vi "MeasureDarkCurrentSimulation.vi"() -> (2 "Amplifier Error":errorcluster)   [LabVIEW 2017]
uses:
  AmplifierSim.lvclass
  MultimeterSim.lvclass
panel:
  out "Final voltage":dbl
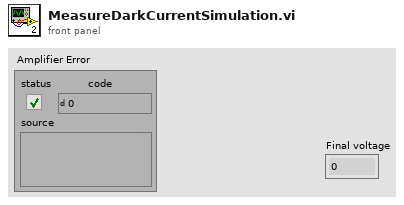
[diagram p1: front panel]
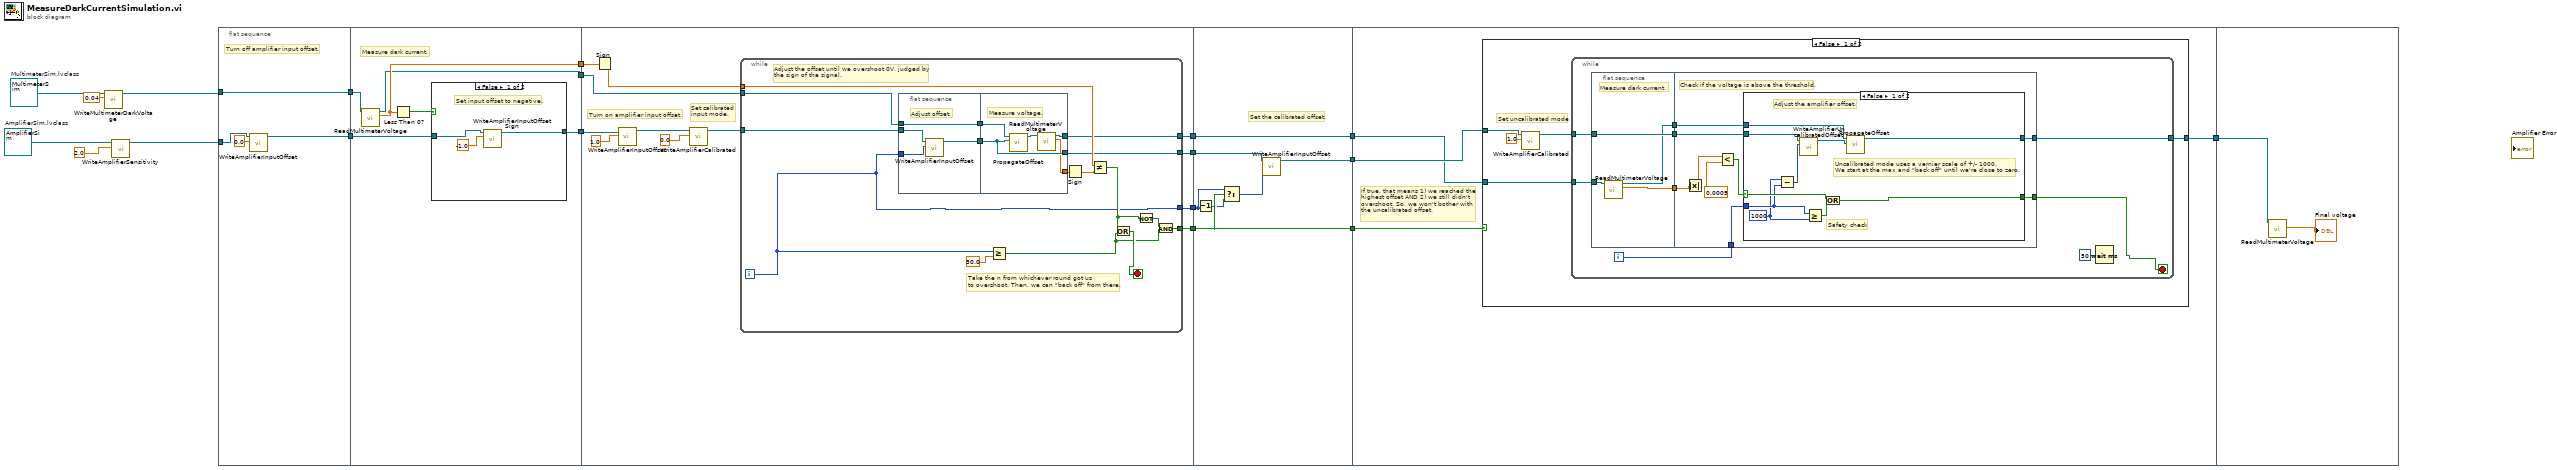
[diagram p0: block diagram]
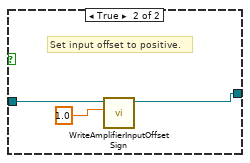
[diagram p2: hidden frame]
diagram:
  w6 = refnum<class "MultimeterSim.lvclass"> refnum  # MultimeterSim.lvclass
  w3 = refnum<class "AmplifierSim.lvclass"> refnum  # AmplifierSim.lvclass
  n1 = call-dynamic "WriteMultimeterDarkVoltage.vi"("Dark Voltage"=0.04, "MultimeterSim in"=w6) -> ("MultimeterSim out"=w5:refnum<class "MultimeterSim.lvclass">)  [unwired: 8 in, 1 out]
  n2 = call-dynamic "WriteAmplifierSensitivity.vi"("Sensitivity"=2.0, "AmplifierSim in"=w3) -> ("AmplifierSim out"=w1:refnum<class "AmplifierSim.lvclass">)  [unwired: 8 in, 1 out]
  n3 = flat-sequence {
    tunnel: w1 -> [w22]
    tunnel: [w21] -> w15
    tunnel: w5 -> [w21]
    tunnel: [w20] -> w14
    tunnel: [w27] -> w19
    tunnel: w15 -> [w28]
    tunnel: w14 -> [w26]
    tunnel: [w25] -> w13
    tunnel: [w24] -> w12
    tunnel: w19 -> [w47]
    tunnel: [w45] -> w18
    tunnel: [w44] -> w16
    tunnel: w13 -> [w43]
    tunnel: w12 -> [w38]
    tunnel: [w37] -> w11
    tunnel: [w36] -> w8
    tunnel: w18 -> [w73]
    tunnel: [w76] -> w17
    tunnel: w16 -> [w76]
    tunnel: w11 -> [w79]
    tunnel: [w78] -> w10
    tunnel: [w77] -> w9
    tunnel: w8 -> [w77]
    tunnel: w17 -> [w83]
    tunnel: w10 -> [w82]
    tunnel: w9 -> [w81]
    tunnel: [w80] -> w7
    tunnel: w7 -> [w122]
    frame #0 {
      # "Turn off amplifier input offset."
      n4 = call-dynamic "WriteAmplifierInputOffset.vi"("Input Offset"=0.0, "AmplifierSim in"=w22) -> ("AmplifierSim out"=w20:refnum<class "AmplifierSim.lvclass">)  [unwired: 8 in, 1 out]
    }
    frame #1 {
      # "Measure dark current."
      n5 = call-dynamic "ReadMultimeterVoltage.vi"("MultimeterSim in"=w28) -> ("Voltage"=w27:dbl, "MultimeterSim out"=w24:refnum<class "MultimeterSim.lvclass">)  [unwired: 8 in, 1 out]
      n6 = Less Than 0?(x=w27) -> (x < 0?=w29:bool)
      n7 = case shown="False" w29 {
        tunnel: w26 -> [w31 w35]
        tunnel: [w30 w33] -> w25
        frame False {
          # "Set input offset to negative."
          n8 = call-dynamic "WriteAmplifierInputOffsetSign.vi"("Input Offset Sign"=-1.0, "AmplifierSim in"=w31) -> ("AmplifierSim out"=w30:refnum<class "AmplifierSim.lvclass">)  [unwired: 8 in, 1 out]
        }
        frame True {
          # "Set input offset to positive."
          n9 = call-dynamic "WriteAmplifierInputOffsetSign.vi"("Input Offset Sign"=1.0, "AmplifierSim in"=w35) -> ("AmplifierSim out"=w33:refnum<class "AmplifierSim.lvclass">)  [unwired: 8 in, 1 out]
        }
      }
    }
    frame #2 {
      # "Set calibrated \ninput mode."
      # "Turn on amplifier input offset."
      n10 = Sign(1:w47) -> (0:w46:dbl)
      n11 = call-dynamic "WriteAmplifierInputOffset.vi"("Input Offset"=1.0, "AmplifierSim in"=w43) -> ("AmplifierSim out"=w40:refnum<class "AmplifierSim.lvclass">)  [unwired: 8 in, 1 out]
      n12 = call-dynamic "WriteAmplifierCalibrated.vi"("Calibrated"=0.0, "AmplifierSim in"=w40) -> ("AmplifierSim out"=w39:refnum<class "AmplifierSim.lvclass">)  [unwired: 8 in, 1 out]
      n13 = while {
        tunnel: w46 -> [w61]
        tunnel: [w48] -> w45
        tunnel: [w56] -> w44
        tunnel: w39 -> [w55]
        tunnel: w38 -> [w53]
        tunnel: [w51] -> w37
        tunnel: [w50] -> w36
        i -> [w48]
        stop <- w60 stop-if-true
        # "Take the n from whichever round got us \nto overshoot. Then, we can \"back off\" from there."
        # "Adjust the offset until we overshoot 0V, judged by\nthe sign of the signal."
        n14 = flat-sequence {
          tunnel: w48 -> [w66]
          tunnel: w55 -> [w67]
          tunnel: [w65] -> w54
          tunnel: w53 -> [w64]
          tunnel: [w64] -> w52
          tunnel: w54 -> [w71]
          tunnel: w52 -> [w72]
          tunnel: [w71] -> w51
          tunnel: [w68] -> w50
          tunnel: [w70] -> w49
          frame #0 {
            # "Adjust offset."
            n15 = call-dynamic "WriteAmplifierInputOffset.vi"("Input Offset"=w66, "AmplifierSim in"=w67) -> ("AmplifierSim out"=w65:refnum<class "AmplifierSim.lvclass">)  [unwired: 8 in, 1 out]
          }
          frame #1 {
            # "Measure voltage."
            n16 = call "PropagateOffset.vi"("AmplifierSim.lvclass"=w71, "MultimeterSim.lvclass"=w72) -> ("MultimeterSimOut"=w69:refnum<class "MultimeterSim.lvclass">)  [unwired: 9 in]
            n17 = call-dynamic "ReadMultimeterVoltage.vi"("MultimeterSim in"=w69) -> ("Voltage"=w70:dbl, "MultimeterSim out"=w68:refnum<class "MultimeterSim.lvclass">)  [unwired: 8 in, 1 out]
          }
        }
        n18 = Greater Or Equal?(x=w48, y=30.0) -> (x >= y?=w57:bool)
        n19 = Sign(1:w49) -> (0:w62:dbl)
        n20 = Not Equal?(x=w61, y=w62) -> (x != y?=w59:bool)
        n21 = Or(x=w59, y=w57) -> (x .or. y?=w60:bool)
        n22 = Not(x=w59) -> (.not. x?=w58:bool)
        n23 = And(x=w58, y=w57) -> (x .and. y?=w56:bool)
      }
    }
    frame #3 {
      # "Set the calibrated offset."
      n24 = Decrement(x=w73) -> (x-1=w74:i32)
      n25 = Select(t=w73, s=w76, f=w74) -> (s? t:f=w75:i32)
      n26 = call-dynamic "WriteAmplifierInputOffset.vi"("Input Offset"=w75, "AmplifierSim in"=w79) -> ("AmplifierSim out"=w78:refnum<class "AmplifierSim.lvclass">)  [unwired: 8 in, 1 out]
    }
    frame #4 {
      # "If true, that means 1) we reached the \nhighest offset AND 2) we still didn't \novershoot. So, we won't bother with \nthe uncalibrated offset."
      n27 = case shown="False" w83 {
        tunnel: w82 -> [w87 _]
        tunnel: w81 -> [w85 _]
        tunnel: [w84 _] -> w80
        frame False {
          # "Set uncalibrated mode"
          n28 = call-dynamic "WriteAmplifierCalibrated.vi"("Calibrated"=1.0, "AmplifierSim in"=w87) -> ("AmplifierSim out"=w86:refnum<class "AmplifierSim.lvclass">)  [unwired: 8 in, 1 out]
          n29 = while {
            tunnel: w86 -> [w92]
            tunnel: w85 -> [w90]
            tunnel: [w89] -> w84
            i -> [w97]
            stop <- w96 stop-if-true
            n30 = flat-sequence {
              tunnel: [w101] -> w94
              tunnel: [w100] -> w93
              tunnel: w92 -> [w100]
              tunnel: [w99] -> w91
              tunnel: w90 -> [w98]
              tunnel: [w107] -> w96
              tunnel: w97 -> [w106]
              tunnel: w94 -> [w105]
              tunnel: w93 -> [w104]
              tunnel: w91 -> [w103]
              tunnel: [w102] -> w89
              frame #0 {
                # "Measure dark current."
                n31 = call-dynamic "ReadMultimeterVoltage.vi"("MultimeterSim in"=w98) -> ("Voltage"=w101:dbl, "MultimeterSim out"=w99:refnum<class "MultimeterSim.lvclass">)  [unwired: 8 in, 1 out]
              }
              frame #1 {
                # "Check if the voltage is above the threshold."
                n32 = Absolute Value(x=w105) -> (abs(x)=w110:dbl)
                n33 = Less?(x=w110, y=0.0005) -> (x < y?=w108:bool)
                n34 = case shown="False" w108 {
                  selector: w108 -> [w119 _]
                  tunnel: [w120 _] -> w107
                  tunnel: w106 -> [w117 _]
                  tunnel: w104 -> [w114 _]
                  tunnel: w103 -> [w112 _]
                  tunnel: [w111 _] -> w102
                  frame False {
                    w116 = 1000
                    # "Safety check"
                    # "Uncalibrated mode uses a vernier scale of +/- 1000. \nWe start at the max and \"back off\" until we're close to zero."
                    # "Adjust the amplifier offset."
                    n35 = Subtract(x=w116, y=w117) -> (x-y=w115:i32)
                    n36 = call-dynamic "WriteAmplifierUncalibratedOffset.vi"("Uncalibrated Offset"=w115, "AmplifierSim in"=w114) -> ("AmplifierSim out"=w113:refnum<class "AmplifierSim.lvclass">)  [unwired: 8 in, 1 out]
                    n37 = Greater Or Equal?(x=w117, y=w116) -> (x >= y?=w118:bool)
                    n38 = Or(x=w119, y=w118) -> (x .or. y?=w120:bool)
                    n39 = call "PropagateOffset.vi"("AmplifierSim.lvclass"=w113, "MultimeterSim.lvclass"=w112) -> ("MultimeterSimOut"=w111:refnum<class "MultimeterSim.lvclass">)  [unwired: 9 in]
                  }
                  frame True {
                  }
                }
              }
            }
            n40 = Wait (ms)(milliseconds to wait=u32 50) -> ()  [unwired: 1 out]
          }
        }
        frame True {
        }
      }
    }
    frame #5 {
      n41 = call-dynamic "ReadMultimeterVoltage.vi"("MultimeterSim in"=w122) -> ("Voltage"=→"Final voltage":dbl)  [unwired: 8 in, 2 out]
    }
  }
